vi "display matrix to spreadsheet string.vi"(8 "error in":errorcluster, 11 "Display":string[][](table)) -> (0 "error out":errorcluster, 1 "num cols":i32, 2 "num rows":i32, 3 "spreadsheet string":string)   [LabVIEW 2018]
uses:
  <vilib>/regexp/Match Regular Expression.xnode
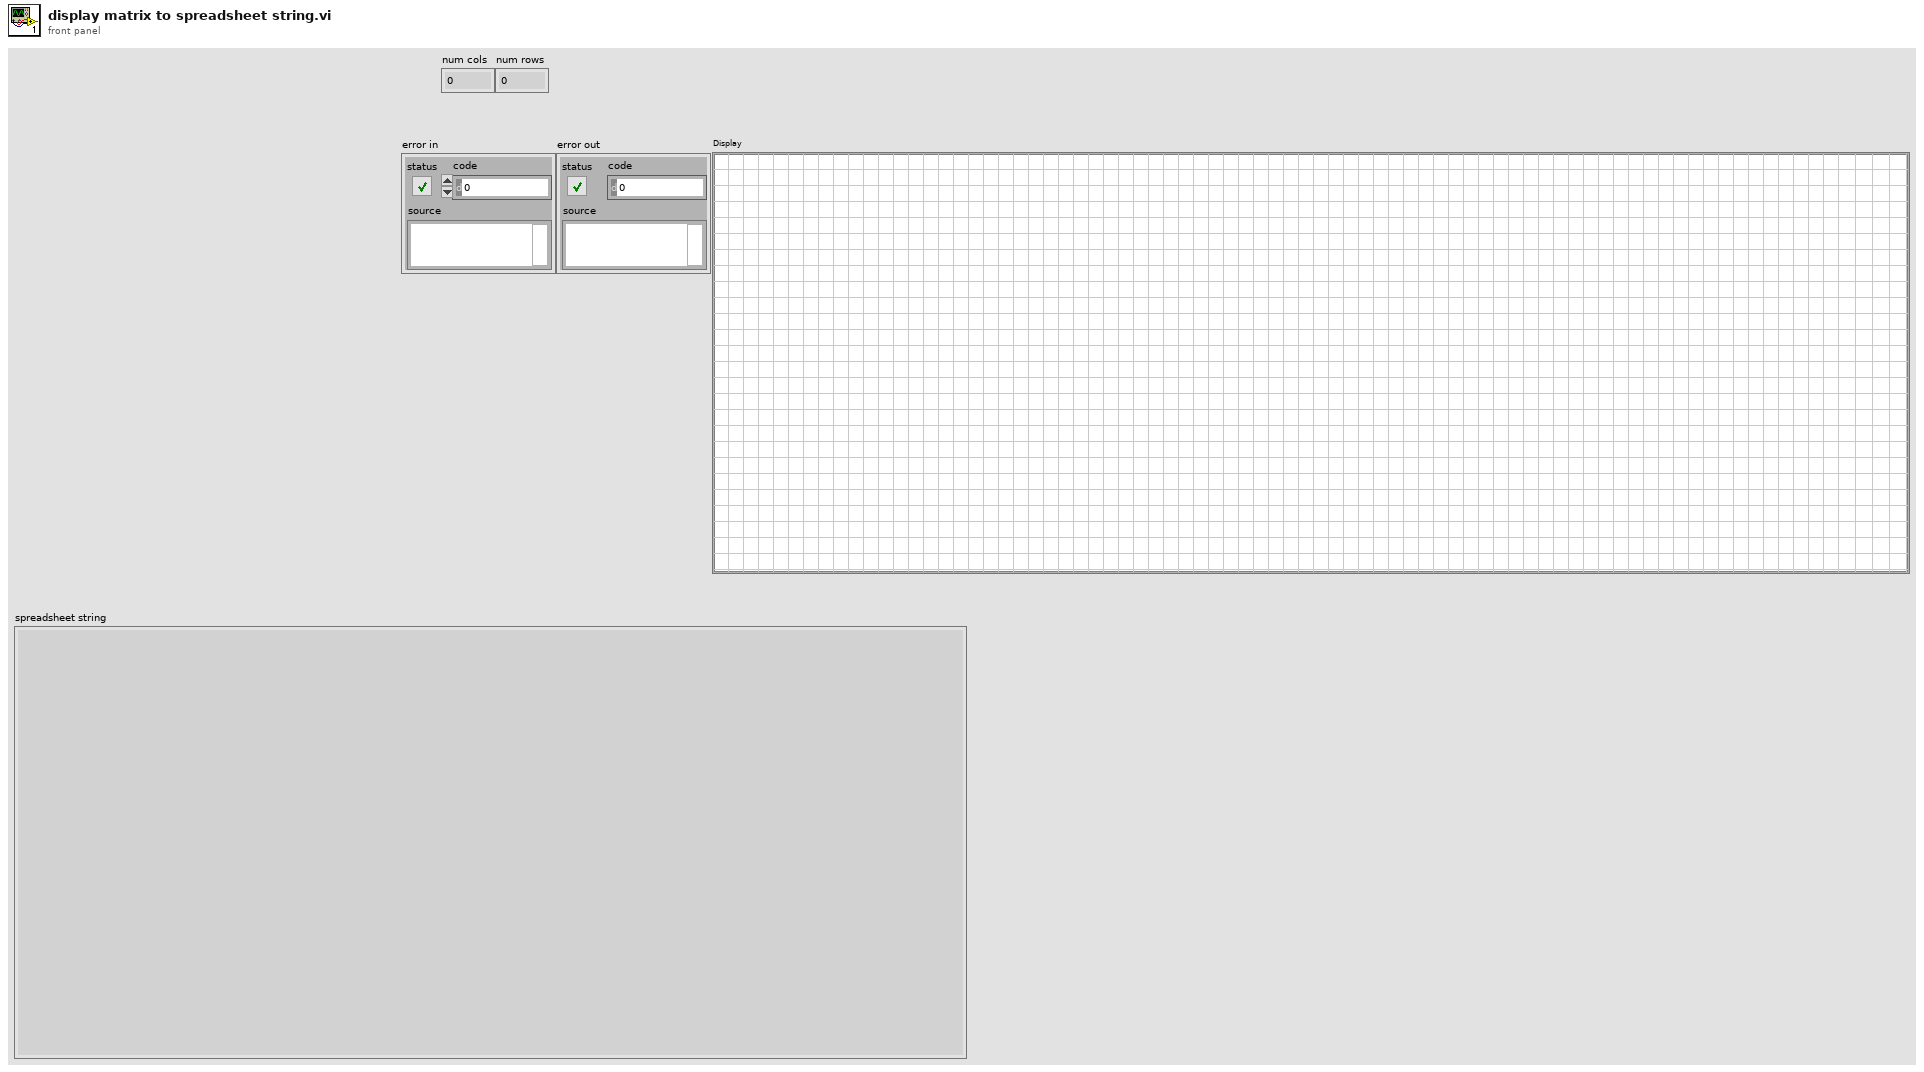
[diagram p1: front panel]
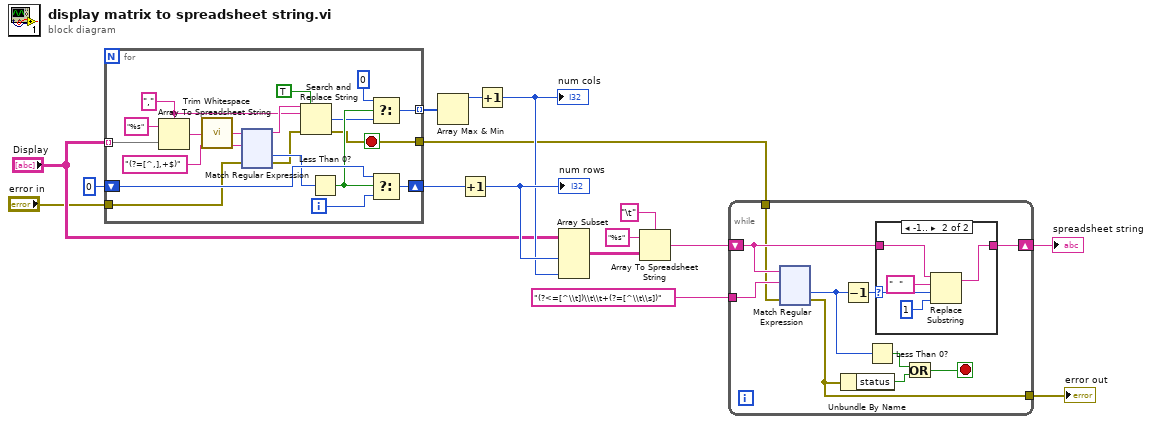
[diagram p0: block diagram]
diagram:
  n1 = for {
    tunnel: "Display" -> [w34] mode=indexing
    tunnel: [w21] -> w14 mode=indexing
    shift-right: [w29] -> w12
    shift-left: 0 -> [w28]
    tunnel: [w18] -> w6
    tunnel: "error in" -> [w17]
    i -> [w30]
    stop <- w18 stop-if-true
    w26 = "," ("delimiter (Tab)")
    n2 = Array To Spreadsheet String(delimiter (Tab)=w26, array=w34, 3:"%s" ("format string")) -> (spreadsheet string=w32:string)
    n3 = call <vilib>:"Trim Whitespace.vi"("string"=w32) -> ("trimmed string"=w31:string)  [unwired: 1 in]
    n4 = xnode "Match Regular Expression"("input string"=w31, "regular expression"="(?=[^,],+$)" ("delimiter (Tab)"), "error in"=w17) -> ("before match"=w27:string, "offset past match"=w24:i32, "error out"=w19:errorcluster)  [unwired: 3 in, 2 out]
    n5 = Search and Replace String(replace all?=TRUE ("replace all? (F)"), input string=w27, search string=w26, error in=w19) -> (number of replacements=w22:i32, error out=w18:errorcluster)  [unwired: 4 in, 2 out]
    n6 = Less Than 0?(x=w24) -> (x < 0?=w23:bool)
    n7 = Select(t=0, s=w23, f=w22) -> (s? t:f=w21:i32)
    n8 = Select(t=w28, s=w23, f=w30) -> (s? t:f=w29:i32)
  }
  n9 = Array Max & Min(array=w14) -> (max value=w10:i32)  [unwired: 3 out]
  n10 = Increment(x=w12) -> (x+1=w11:i32)
  "num rows" <- w11
  n11 = Increment(x=w10) -> (x+1=w9:i32)
  "num cols" <- w9
  n12 = Array Subset(array="Display", length (row)=w11, length (col)=w9) -> (w8:string[][])  [unwired: 2 in]
  n13 = Array To Spreadsheet String(delimiter (Tab)="\t", array=w8, 3:"%s" ("format string")) -> (spreadsheet string=w7:string)
  n14 = while {
    shift-right: [w155] -> w3
    shift-left: w7 -> [w156]
    tunnel: "(?<=[^\\t])\\t\\t+(?=[^\\t\\s])" ("format string") -> [w152]
    tunnel: [w148] -> w4
    tunnel: w6 -> [w147]
    stop <- w149 stop-if-true
    n15 = xnode "Match Regular Expression"("input string"=w156, "regular expression"=w152, "error in"=w147) -> ("offset past match"=w154:i32, "error out"=w148:errorcluster)  [unwired: 3 in, 3 out]
    n16 = Unbundle By Name(w148) -> ("status"=w150:bool)
    n17 = Decrement(x=w154) -> (x-1=w153:i32)
    n18 = Less Than 0?(x=w154) -> (x < 0?=w151:bool)
    n19 = case shown="-1.." w153 {
      selector: w153 -> [_ w158]
      tunnel: w156 -> [w157 w162]
      tunnel: [w157 w159] -> w155
      frame Default {
      }
      frame -1.. {
        n20 = Replace Substring(2:1 ("length (len. of substring)"), 3:w158, 4:"  " ("substring (\"\")"), 5:w162) -> (1:w159:string)  [unwired: 1 out]
      }
    }
    n21 = Or(x=w151, y=w150) -> (x .or. y?=w149:bool)
  }
  "spreadsheet string" <- w3
  "error out" <- w4
